vi "voice.vi"() -> ()   [LabVIEW 2012]
uses:
  <vilib>/sound2/lvsound2.llb/Sampling Mode.ctl
  <vilib>/sound2/lvsound2.llb/Sound Data Format.ctl
  <vilib>/sound2/lvsound2.llb/Sound Input Read (DBL).vi
  <vilib>/Analysis/3filter.llb/Butterworth Filter (DBL).vi
  <vilib>/measure/matone.llb/Extract Single Tone Information 1 Chan.vi
  <vilib>/Analysis/NI_AALBase.lvlib
  <vilib>/measure/NI_MAPro.lvlib
panel:
  in  "x 2":dbl
  in  "y 2":dbl
  out "要对比声音波形":dynamicdata(graph)
  out "原始波形":dynamicdata(graph)
  in  "sound format":T1={"sample rate (S/s)"=22050.0, "number of channels"=2, "bits per sample"=16} caption="声音格式"
  in  "device ID":u32 caption="设备ID"
  in  "sample mode":T2=1 caption="采样模式" items=["有限采样", "连续采样"]
  in  "number of samples/ch":i32=100000 caption="每通道采样数"
  out "error out":errorcluster caption="错误输出"
  out "波形存储":dynamicdata(graph)
  in  "停止1":bool
  in  "Lower Cut-Off":dbl=60.0 caption="低截止频率"
  in  "Upper Cut-Off":dbl=2500.0 caption="高截止频率"
  in  "Filename":path=path "C:/Users/Administrator/Desktop/1.lvm" caption="波形保存路径"
  in  "停止 2":bool
  in  "x":dbl
  in  "y":dbl
  out "指示灯":bool
  in  "选择":enum16{"波形存储", "波形对比识别"}(ring)
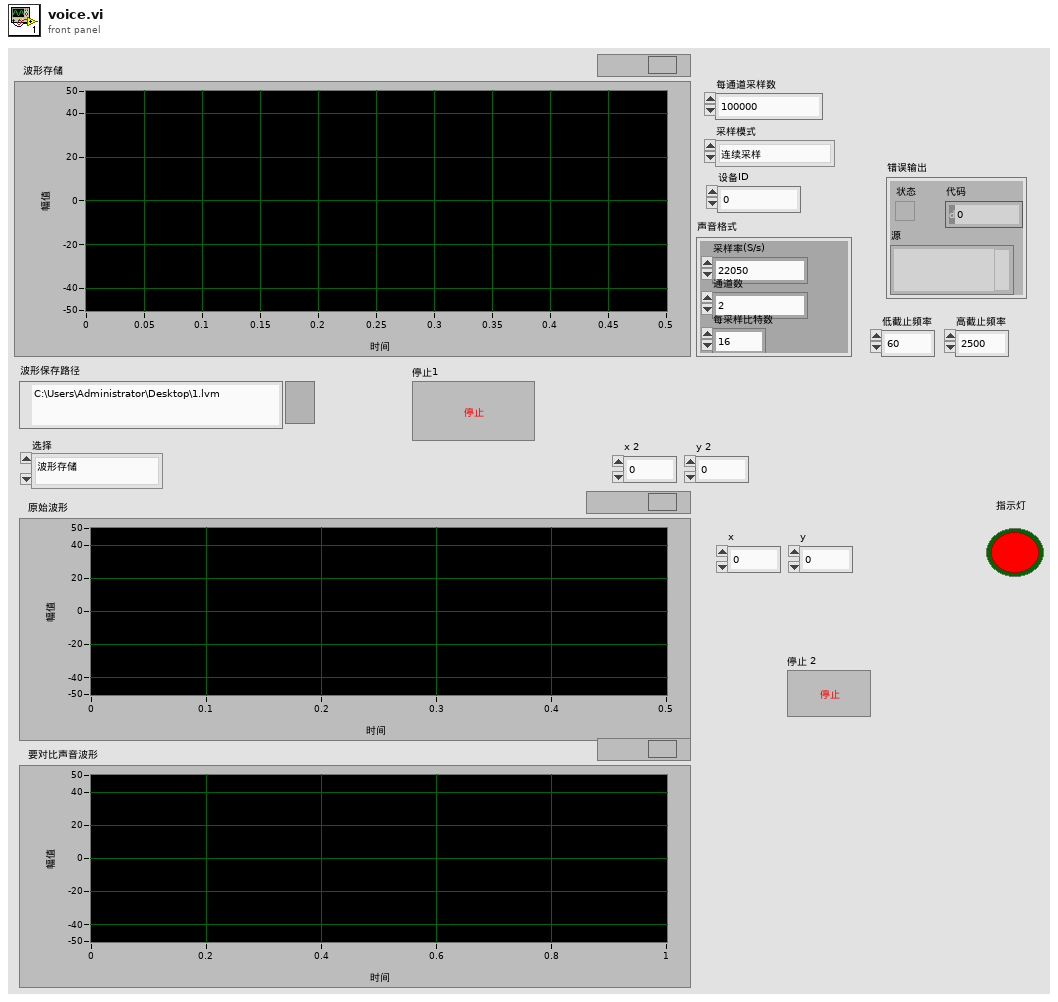
[diagram p1: front panel]
types:
  T1 = typedef "Sound Data Format.ctl" = cluster{"sample rate (S/s)":dbl, "number of channels":i32, "bits per sample":i32}
  T2 = typedef "Sampling Mode.ctl" = i32
  T3 = typedef "Sound Input Task ID.ctl" = u32
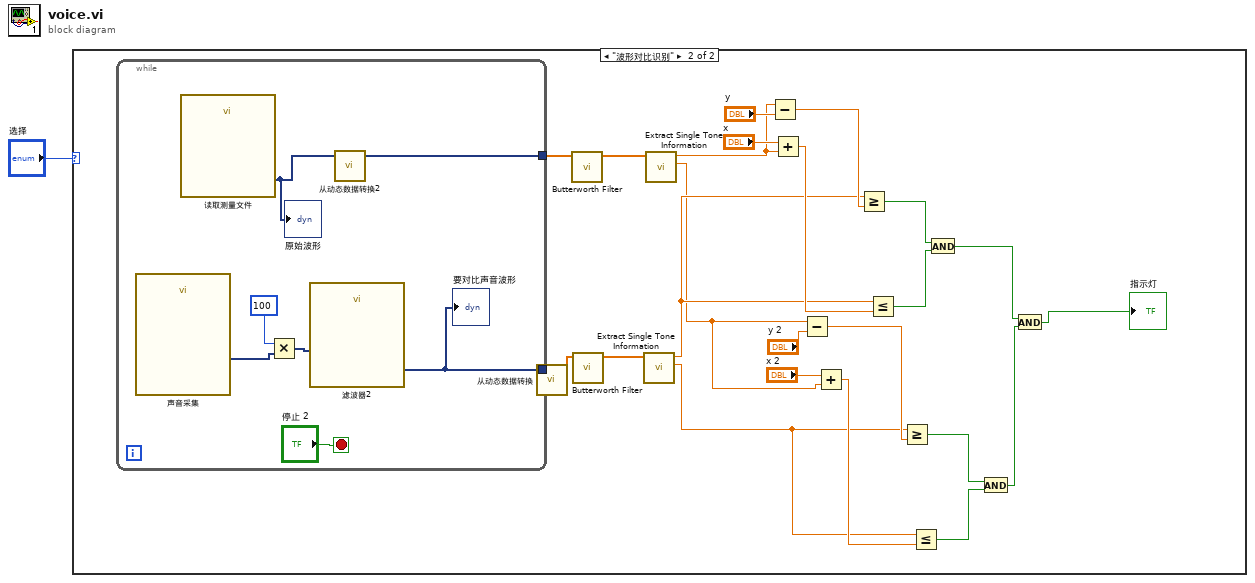
[diagram p0: block diagram]
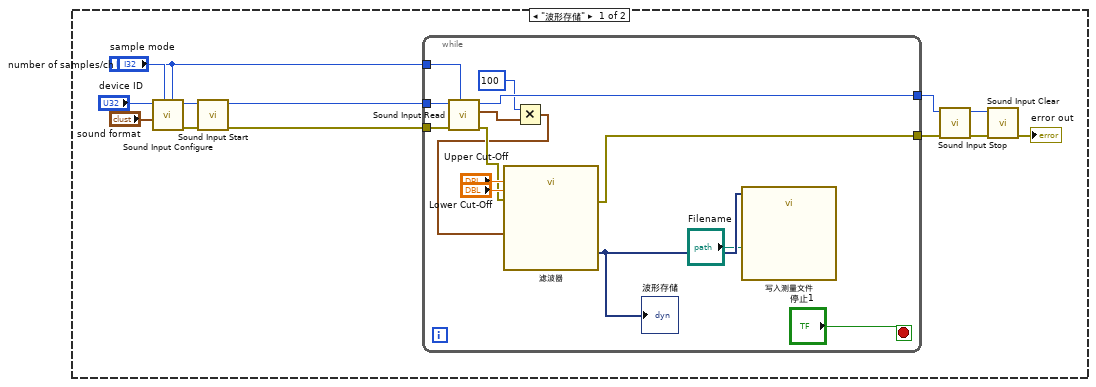
[diagram p2: hidden frame]
diagram:
  n1 = case shown="\"波形对比识别\"" "选择" {
    frame "波形存储" {
      n2 = call <vilib>:"Sound Input Configure.vi"("number of samples/ch"="number of samples/ch", "sample mode"="sample mode", "sound format"="sound format", "device ID"="device ID") -> ("error out"=w14:errorcluster, "task ID"=w13:T3)  [unwired: 6 in]
      n3 = call <vilib>:"Sound Input Start.vi"("error in (no error)"=w14, "task ID"=w13) -> ("error out"=w11:errorcluster, "task ID out"=w12:T3)  [unwired: 8 in]
      n4 = while {
        tunnel: w12 -> [w28]
        tunnel: w11 -> [w27]
        tunnel: "number of samples/ch" -> [w25]
        tunnel: [w24] -> w3
        tunnel: [w21] -> w2
        stop <- "停止1" stop-if-true
        n5 = call-poly <vilib>:"Sound Input Read.vi"("number of samples/ch"=w25, "error in (no error)"=w27, "task ID"=w28) -> ("error out"=w20:errorcluster, "data"=w19:waveform(dbl)[], "task ID out"=w24:T3)  [unwired: 6 in]
        n6 = Multiply(x=100, y=w19) -> (x*y=w18:waveform(dbl)[])
        n7 = call "滤波器"("error in (no error)"=w20, "Lower Cut-Off"="Lower Cut-Off", "Upper Cut-Off"="Upper Cut-Off", "Signal"=w18) -> ("error out"=w21:errorcluster, "Filtered Signal"=w16:dynamicdata)  [unwired: 6 in]
        "波形存储" <- w16
        n8 = call "写入测量文件"("Signals"=w16, "Filename"="Filename") -> ()  [unwired: 15 in, 3 out]
      }
      n9 = call <vilib>:"Sound Input Stop.vi"("error in (no error)"=w2, "task ID"=w3) -> ("error out"=w10:errorcluster, "task ID out"=w9:T3)  [unwired: 8 in]
      n10 = call <vilib>:"Sound Input Clear.vi"("error in (no error)"=w10, "task ID"=w9) -> ("error out"=→"error out":errorcluster)  [unwired: 9 in]
    }
    frame "波形对比识别" {
      n11 = while {
        tunnel: [w58] -> w43
        tunnel: [w54] -> w41
        stop <- "停止 2" stop-if-true
        n12 = call "声音采集"() -> ("Data"=w56:dynamicdata)  [unwired: 18 in, 1 out]
        n13 = call "读取测量文件"() -> ("Signals"=w58:dynamicdata)  [unwired: 6 in, 5 out]
        "原始波形" <- w58
        n14 = Multiply(x=100, y=w56) -> (x*y=w55:dynamicdata)
        n15 = call "滤波器2"("Signal"=w55) -> ("Filtered Signal"=w54:dynamicdata)  [unwired: 9 in, 1 out]
        "要对比声音波形" <- w54
      }
      n16 = call "从动态数据转换2"("Dynamic Data Type"=w43) -> ("Array"=w42:dbl[])  [unwired: 3 in]
      n17 = call "从动态数据转换"("Dynamic Data Type"=w41) -> ("Array"=w40:dbl[])  [unwired: 3 in]
      n18 = call-poly <vilib>:"Butterworth Filter.vi"("X"=w42) -> ("Filtered X"=w53:dbl[])  [unwired: 7 in, 1 out]
      n19 = call-poly <vilib>:"Butterworth Filter.vi"("X"=w40) -> ("Filtered X"=w52:dbl[])  [unwired: 7 in, 1 out]
      n20 = call-poly <vilib>:"Extract Single Tone Information.vi"("time signal in"=w52) -> ("detected amplitude"=w32:dbl, "detected frequency"=w46:dbl)  [unwired: 5 in, 4 out]
      n21 = call-poly <vilib>:"Extract Single Tone Information.vi"("time signal in"=w53) -> ("detected amplitude"=w33:dbl, "detected frequency"=w49:dbl)  [unwired: 5 in, 4 out]
      n22 = Subtract(x=w49, y="y") -> (x-y=w48:dbl)
      n23 = Add(x="x", y=w49) -> (x+y=w47:dbl)
      n24 = Subtract(x=w33, y="y 2") -> (x-y=w37:dbl)
      n25 = Add(x="x 2", y=w33) -> (x+y=w36:dbl)
      n26 = Greater Or Equal?(x=w46, y=w48) -> (x >= y?=w45:bool)
      n27 = Less Or Equal?(x=w46, y=w47) -> (x <= y?=w44:bool)
      n28 = Greater Or Equal?(x=w32, y=w37) -> (x >= y?=w34:bool)
      n29 = Less Or Equal?(x=w32, y=w36) -> (x <= y?=w35:bool)
      n30 = And(x=w45, y=w44) -> (x .and. y?=w30:bool)
      n31 = And(x=w34, y=w35) -> (x .and. y?=w31:bool)
      n32 = And(x=w30, y=w31) -> (x .and. y?=→"指示灯":bool)
    }
  }
